vi "PMA Messdatenverteiler.vi"(8 "error IO":errorcluster) -> (0 "error IO":errorcluster)   [LabVIEW 2020, in "ABB-EL3000.lvlib" / "PMA.lvlib"]
uses:
  PMA.lvlib
  Allgemeine VI/FGV Uras26 Aktion.ctl
  FT-IR/FGV FT-IR Aktionen.ctl
  Status Analysatoren/Aktion Status Analysatoren.ctl
  Allgemeine VI/Aktion FGV Werte Standardanalysator.ctl
  Aktion FGV Messwerte.ctl
  Kalibrieren/Kalibrieren.lvlib
  Allgemeine VI/Allgemeine VI.lvlib
  FT-IR/FT-IR.lvlib
  Status Analysatoren/Status Analysatoren.lvlib
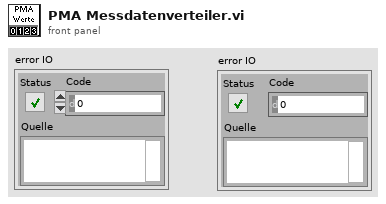
[diagram p1: front panel]
types:
  T1 = typedef "ABB-EL3000.lvlib/Allgemeine VI.lvlib/FGV Uras26 Aktion.ctl" = enum16{"lesen", "CAL-Daten laden", "Messen", "Kalibrieren vorbereiten", "Kalibrieren", "CAL-Daten speichern", "Toleranz schreiben", "CAL-Daten kopieren"}
  T2 = typedef "ABB-EL3000.lvlib/Allgemeine VI.lvlib/Aktion FGV Werte Standardanalysator.ctl" = enum16{"lesen", "FID", "PMA"}
  T3 = typedef "Status Analysatoren.lvlib/Aktion Status Analysatoren.ctl" = enum16{"lesen", "initialisieren", "Analysatoren aktiv", "FTIR Fehler", "FID Fehler", "PMA Fehler", "Felder einfärben"}
  T4 = typedef "FT-IR.lvlib/FGV FT-IR Aktionen.ctl" = enum16{"lesen", "NOG setzen", "NOS setzen", "Initialisieren", "speichern", "ALLES setzen", "FT-IR Spektrum loggen", "Komm Stoppen", "Spektrum LogKonfig"}
  T5 = typedef "ABB-EL3000.lvlib/PMA.lvlib/Aktion FGV Messwerte.ctl" = enum16{"lesen", "Messwerte", "Messbereich", "Status", "Diagnose Werte"}
  T6 = typedef "Status Analysatoren.lvlib/Status.ctl" = cluster{"FT-IR aktiv":bool, "FT-IR Fehler":bool, "FID aktiv":bool, "FID Fehler":bool, "PMA aktiv":bool, "PMA Fehler":bool}
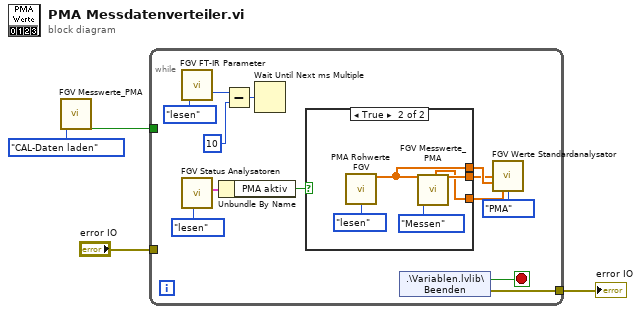
[diagram p0: block diagram]
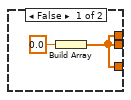
[diagram p2: hidden frame]
diagram:
  n1 = call "FGV Messwerte_PMA.vi"("Aktion"=FGV_Uras26_Aktion."CAL-Daten laden") -> ("CAL TimeOut"=w1:bool)  [unwired: 19 in, 7 out]
  n2 = while {
    tunnel: [w16] -> w4
    tunnel: "error IO" -> [_]
    tunnel: w1 -> [_]
    stop <- w17 stop-if-true
    n3 = call "FGV FT-IR Parameter.vi"("Aktion"=FGV_FT-IR_Aktionen."lesen") -> ("Zykluszeit Messdatenverteiler"=w14:u32)  [unwired: 11 in, 7 out]
    n4 = call "FGV Status Analysatoren.vi"("Aktionen"=Aktion_Status_Analysatoren."lesen") -> ("Status Analysatoren"=w11:T6)  [unwired: 10 in]
    n5 = Unbundle By Name(w11) -> ("PMA aktiv"=w9:bool)
    n6 = Subtract(x=w14, y=u32 10) -> (x-y=w13:u32)
    n7 = Wait Until Next ms Multiple(millisecond multiple=w13) -> ()  [unwired: 1 out]
    n8 = case shown="True" w9 {
      tunnel: [w18 w22] -> w7
      tunnel: [w18 w21] -> w8
      tunnel: [w18 w20] -> w5
      frame False {
        n9 = Build Array(sgl 0.0 ("Element")) -> (w18:sgl[])
      }
      frame True {
        n10 = call "PMA Rohwerte FGV.vi"("Aktion"=Aktion_FGV_Messwerte."lesen") -> ("Messwerte"=w21:sgl[])  [unwired: 11 in, 3 out]
        n11 = call "FGV Messwerte_PMA.vi"("GasValue"=w21, "Aktion"=FGV_Uras26_Aktion."Messen") -> ("Rohwerte LIN"=w20:sgl[], "GasValue"=w22:sgl[])  [unwired: 18 in, 6 out]
      }
    }
    n12 = shared-variable ".\\Variablen.lvlib\\Beenden"() -> (w17:bool, error out=w16:errorcluster)  [unwired: 1 in]
    n13 = call "FGV Werte Standardanalysator.vi"("PMA"=w7, "PMA Rohwerte"=w8, "PMA Rohwert LIN"=w5, "Aktion"=Aktion_FGV_Werte_Standardanalysator."PMA") -> ()  [unwired: 5 in, 7 out]
  }
  "error IO" <- w4
